vi "Colors and buttons example.vi"() -> ()   [LabVIEW 2018]
panel:
  in  "Blank Button 2":bool
  in  "Color Box 4":u32(colorbox)
  in  "Color Box 3":u32(colorbox)
  in  "Color Box 2":u32(colorbox)
  in  "Color Box":u32(colorbox)
  out "Colors [4]":cluster{u32, u32}[](array[cluster])
  out "B":u8
  out "G":u8
  out "Resolved Color":u32 format="%.0x"
  in  "Color":u32(colorbox)
  in  "Boolean":bool
  in  "stop":bool
  out "Blank Button":bool
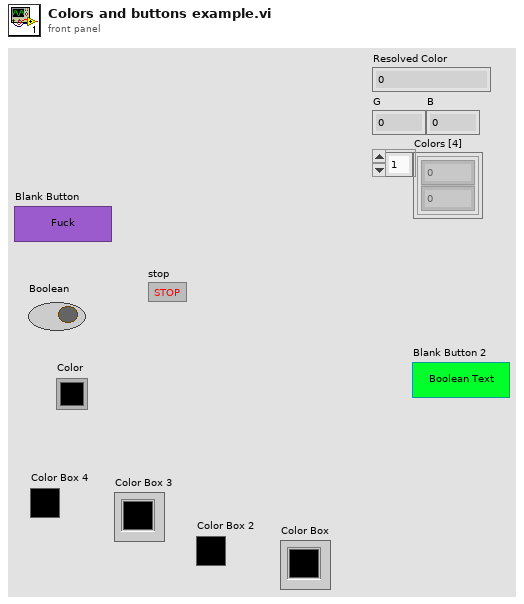
[diagram p1: front panel]
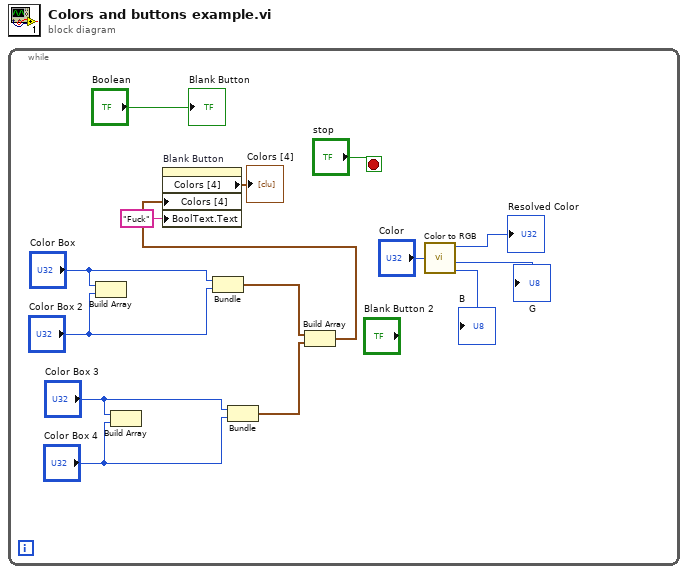
[diagram p0: block diagram]
diagram:
  n1 = while {
    stop <- "stop" stop-if-true
    n2 = Build Array("Color Box", "Color Box 2") -> ()  [unwired: 1 out]
    n3 = Build Array("Color Box 3", "Color Box 4") -> ()  [unwired: 1 out]
    n4 = Bundle("Color Box"="Color Box", "Color Box 2"="Color Box 2") -> (w3:cluster{"Color Box":u32, "Color Box 2":u32})  [unwired: 1 in]
    n5 = Bundle("Color Box 3"="Color Box 3", "Color Box 4"="Color Box 4") -> (w4:cluster{"Color Box 3":u32, "Color Box 4":u32})  [unwired: 1 in]
    n6 = Build Array(w3, w4) -> (w2:cluster{"Color Box 3":u32, "Color Box 4":u32}[])
    n7 = property on="Blank Button" class="Bool"("Colors [4]"=w2, "BoolText.Text"="Fuck" ("Boolean Text.Text")) -> ("Colors [4]"=→"Colors [4]":cluster{u32, u32}[])  [unwired: 2 in, 2 out]
    n8 = call <vilib>:"Color to RGB.vi"("Color"="Color") -> ("Resolved Color"=→"Resolved Color":u32, "G"=→"G":u8, "B"=→"B":u8)  [unwired: 1 out]
    "Blank Button" <- "Boolean"
  }
